vi "FirePneumaticHandler.vi"(0 "MainQueue":refnum<queue>, 5 "cQuickShoot":bool, 7 "cLauncherWheel":bool, 9 "cFirePneumatic":bool, 11 "error in (no error)":errorcluster) -> (15 "error out":errorcluster)   [LabVIEW 2013]
doc: "Takes the button value for FirePneumatic and determines if it has changed. If it has, enqueues an instruction."
uses:
  QueueInstruction.ctl
  SubsystemEnum.ctl
  ActionEnum.ctl
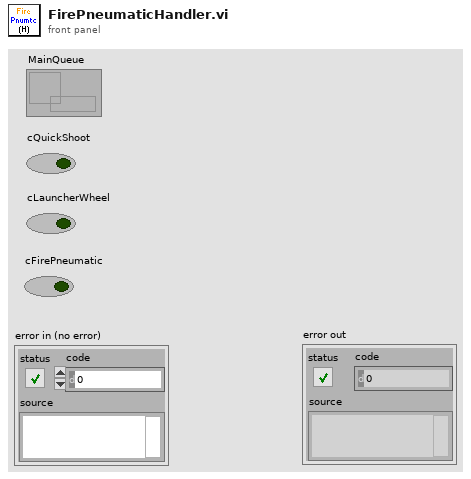
[diagram p1: front panel]
types:
  T1 = typedef "SubsystemEnum.ctl" = enum16{"TankDrive", "FirePneumatic", "Climber", "ClimbWeight", "ShooterAngle"}
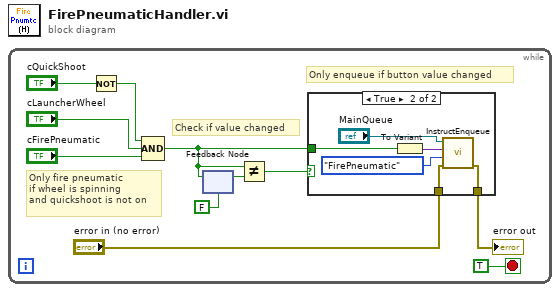
[diagram p0: block diagram]
diagram:
  n1 = while {
    stop <- TRUE stop-if-true
    # "Check if value changed"
    # "Only enqueue if button value changed"
    # "Only fire pneumatic\nif wheel is spinning\nand quickshoot is not on"
    n2 = Not(x="cQuickShoot") -> (.not. x?=w5:bool)
    n3 = Compound Arithmetic op=AND(w5, "cLauncherWheel", "cFirePneumatic") -> (w6:bool)
    n4 = feedback #1(FALSE) -> (w2:bool)
    n5 = feedback-in #1(w6) -> ()
    n6 = Not Equal?(x=w6, y=w2) -> (x != y?=w9:bool)
    n7 = case shown="True" w9 {
      tunnel: w6 -> [_ w18]
      tunnel: "error in (no error)" -> [w12 w14]
      tunnel: [w12 w13] -> w7
      frame False {
      }
      frame True {
        n8 = To Variant(anything=w18) -> (Variant=w16:variant)
        n9 = call "InstructEnqueue.vi"("error in (no error)"=w14, "Subsystem"=SubsystemEnum."FirePneumatic", "Variant"=w16, "Queue"="MainQueue") -> ("error out"=w13:errorcluster)  [unwired: 7 in]
      }
    }
    "error out" <- w7
  }
